vi "create will message.vi"(2 "client?":bool, 3 "subsystem":string) -> (0 "JSON string":string)   [LabVIEW 2017]
uses:
  mqtt client server id.ctl
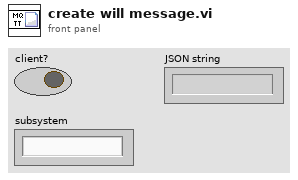
[diagram p1: front panel]
types:
  T1 = typedef "mqtt client server id.ctl" = cluster{"hostname":string, "pid":u32, "state":string, "subsystem":string, "starttime":dbl}
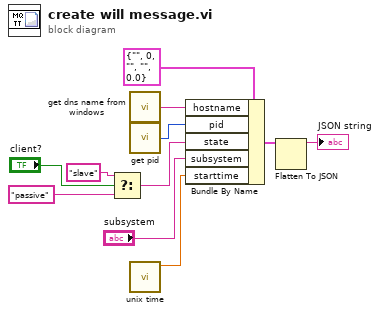
[diagram p0: block diagram]
diagram:
  n1 = Select(t="slave" ("state"), s="client?", f="passive" ("state")) -> (s? t:f=w4:string)
  n2 = call "get dns name from windows.vi"() -> ("ToString"=w2:string)  [unwired: 1 in]
  n3 = call "get pid.vi"() -> ("PID"=w3:u32)  [unwired: 1 in]
  n4 = call "unix time.vi"() -> ("Unix time"=w6:dbl)  [unwired: 10 in, 1 out]
  n5 = Bundle By Name(cluster=T1 {"hostname"="", "pid"=0, "state"="", "subsystem"="", "starttime"=0.0}, "hostname"=w2, "pid"=w3, "state"=w4, "subsystem"="subsystem", "starttime"=w6) -> (w1:T1)
  n6 = Flatten To JSON(anything=w1) -> (JSON string=→"JSON string":string)  [unwired: 2 in, 1 out]
